vi "InputData.vi"(8 "error in (no error)":errorcluster, 10 "clEvtReportArray in":T1 {"Synx" format="%#_4g"}, 11 "ModuleID":i32) -> (0 "error out":errorcluster)   [LabVIEW 2014, in "AppModule.lvlib"]
uses:
  AppModule.lvlib
  Modules/EventPlugins/EventPluginBaseClass/TypeDefs/clEvtReportArray.ctl
  Modules/EventPlugins/EventPluginBaseClass/TypeDefs/clEvtReport.ctl
  clEventType.ctl
  Modules/EventPlugins/EventPluginBaseClass/EventPluginBaseClass.lvclass
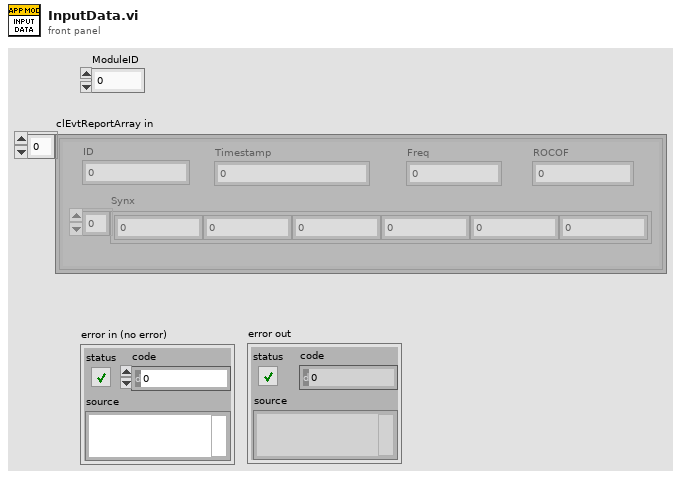
[diagram p1: front panel]
types:
  T1 = typedef "EventPlugins.lvlib/EventPluginBaseClass.lvclass/clEvtReportArray.ctl" = T2[]
  T2 = typedef "EventPlugins.lvlib/EventPluginBaseClass.lvclass/clEvtReport.ctl" = cluster{"Timestamp":dbl, "Synx":cdb[], "Freq":dbl, "ROCOF":dbl, "ID":i16}
  T3 = typedef "AppModule.lvlib/clEventType.ctl" = cluster{"ModuleID":i32, "Data":variant}
  T4 = typedef "AppModule.lvlib/clBroadcastEvents.ctl" = cluster{"DidInit":refnum<user-event>, "StatusUpdate":refnum<user-event>, "ErrorReport":refnum<user-event>, "DidStop":refnum<user-event>, "PathToINI":refnum<user-event>, "InputData":refnum<user-event>, "OutputData":refnum<user-event>, "BcAppInfo":refnum<user-event>, "ConfigData":refnum<user-event>}
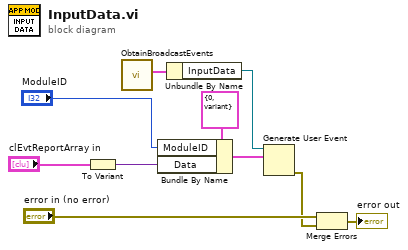
[diagram p0: block diagram]
diagram:
  n1 = To Variant(anything="clEvtReportArray in") -> (Variant=w9:variant)
  n2 = call "ObtainBroadcastEvents.vi"() -> ("AppModuleBroadcast"=w7:T4)  [unwired: 10 in, 1 out]
  n3 = Bundle By Name(cluster=T3 {"ModuleID"=0, "Data"=variant} ("clEventType"), "ModuleID"="ModuleID", "Data"=w9) -> (w6:T3)
  n4 = Unbundle By Name(w7) -> ("InputData"=w5:refnum<user-event>)
  n5 = Generate User Event(user event=w5, event data cluster=w6) -> (error out=w2:errorcluster)  [unwired: 2 in, 1 out]
  n6 = Merge Errors("error in (no error)", w2) -> (→"error out":errorcluster)
